vi "oax_gsLoad Shaft Centerline Data.vi"(11 "data type":i32(listbox)) -> (0 "error out":errorcluster, 1 "end position":i32, 2 "current position":i32, 3 "refnum":refnum<file>, 4 "channel info":T1[](array[typedef]) {"pregain" format="%.2f"; "weighting filter" items=["Linear", "A-weighting", "B-weighting", "C-weighting", "ITU-R 468-4", "Dolby", "CCITT", "C-message", "Wb", "Wc", "Wd", "We", "Wf", "Wh", "Wj", "Wk", "Wm", "AES17 20 kHz lowpass", "AES17 40 kHz lowpass", "AES17 20 kHz highpass", "AES17 40 kHz highpass"]; "dB reference" format="%^.1e"; "engineering units" items=["custom..."=0, "V"=1, "A"=21, "C"=30, "pC"=31, "s"=32, "-"=29, "Pa"=2, "N"=20, "g"=3, "m/s^2"=4, "m/s"=5, "m"=6, "mm/s"=12, "mm"=13, "micron/s"=14, "micron"=15, "in/s^2"=7, "in/s"=8, "in"=9, "mil/s"=10, "mil"=11, "rad/s^2"=16, "rad/s"=17, "rad"=18, "deg/s^2"=26, "deg/s"=27, "deg"=28, "RPM"=22, "cycle/s^2"=23, "Hz"=24, "cycle"=25, "strain"=19]; "sensor sensitivity" format="%#_5f"}, 5 "channel name":string[](array[string]), 6 "pulse / rev":i32)   [LabVIEW 2017]
uses:
  <vilib>/addons/_NISVFA/_Shared subVIs/Controls/svc_Channel Info.ctl
  <vilib>/addons/_NISVFA/_Shared subVIs/Controls/svc_Engineering Units Text Ring.ctl
  <vilib>/addons/_NISVFA/_Shared subVIs/Controls/svc_Weighting Filter Text Ring.ctl
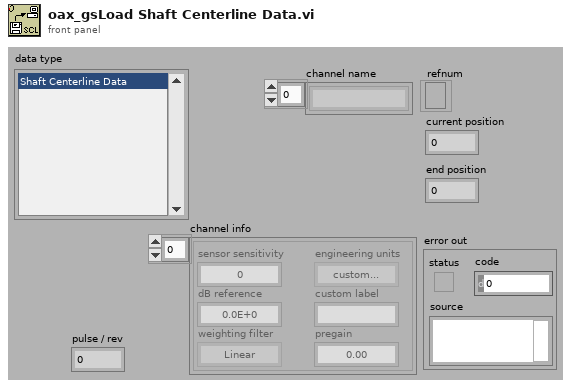
[diagram p1: front panel]
types:
  T1 = typedef "svc_Channel Info.ctl" = cluster{"sensor sensitivity":dbl, "engineering units":T2, "dB reference":dbl, "custom label":string, "weighting filter":T3, "pregain":dbl}
  T2 = typedef "svc_Engineering Units Text Ring.ctl" = u16
  T3 = typedef "svc_Weighting Filter Text Ring.ctl" = u16
  T4 = enum16{"open", "open or create", "create or replace", "create", "open (read only)"}
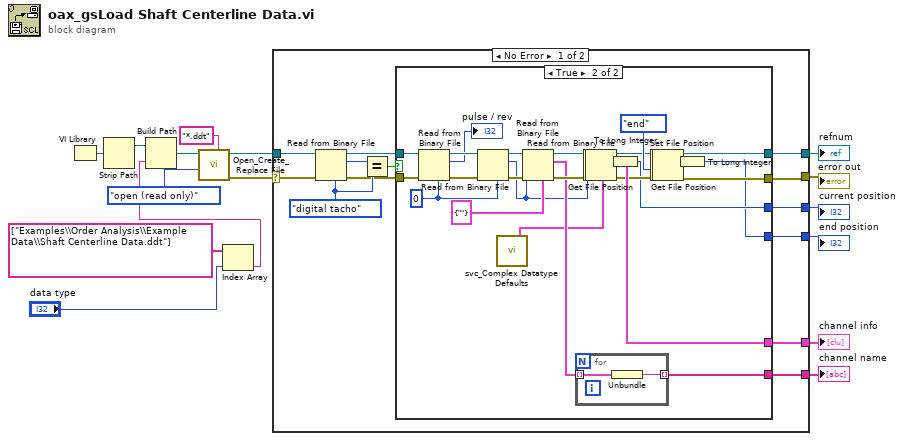
[diagram p0: block diagram]
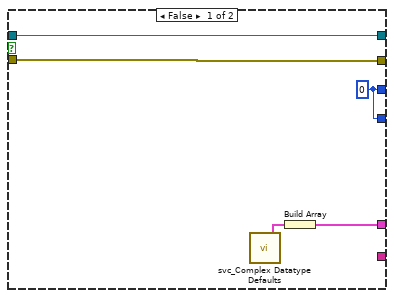
[diagram p2: hidden frame]
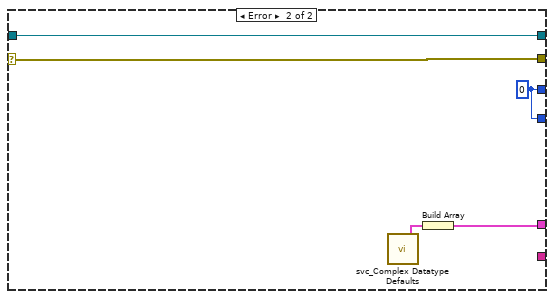
[diagram p3: hidden frame]
diagram:
  n1 = VI Library() -> (path=w14:path)
  n2 = Strip Path(path=w14) -> (stripped path=w13:path)  [unwired: 1 out]
  n3 = Index Array(array=string[] ["Examples\\Order Analysis\\Example Data\\Shaft Centerline Data.ddt"], index="data type") -> (element=w1:string)
  n4 = Build Path(base path=w13, name or relative path=w1) -> (appended path=w12:path)
  n5 = call <vilib>:"Open_Create_Replace File.vi"("pattern"="*.ddt", "function (open:0)"=T4."open (read only)", "file path"=w12) -> ("error out"=w10:errorcluster, "refnum"=w11:refnum<file>)  [unwired: 5 in, 2 out]
  n6 = case shown="No Error" w10 {
    selector: w10 -> [w25 w70]
    tunnel: [w19 w70] -> w8
    tunnel: w11 -> [w29 w69]
    tunnel: [w20 w69] -> w9
    tunnel: [w22 w67] -> w5
    tunnel: [w21 _] -> w4
    tunnel: [w18 w66] -> w7
    tunnel: [w17 w66] -> w6
    frame No Error {
      w27 = enum16{"analog tacho", "digital tacho"}."digital tacho"
      n7 = Read from Binary File(5:w27, 8:w25, 11:w29) -> (0:w23:errorcluster, 2:w28:enum16{"analog tacho", "digital tacho"}, 3:w24:refnum<file>)  [unwired: 3 in, 1 out]
      n8 = Equal?(x=w28, y=w27) -> (x = y?=w26:bool)
      n9 = case shown="True" w26 {
        tunnel: w24 -> [w34 w62]
        tunnel: w23 -> [w33 w63]
        tunnel: [w31 w51] -> w22
        tunnel: [_ w55] -> w21
        tunnel: [w34 w44] -> w20
        tunnel: [w33 w43] -> w19
        tunnel: [w30 w42] -> w18
        tunnel: [w30 w41] -> w17
        frame False {
          w30 = 0 ("offset")
          n10 = call <vilib>:"svc_Complex Datatype Defaults.vi"() -> ("channel info"=w32:T1)  [unwired: 11 in, 8 out]
          n11 = Build Array(w32) -> (w31:T1[])
        }
        frame True {
          w50 = 0
          n12 = Read from Binary File(5:w50, 8:w63, 11:w62) -> (0:w59:errorcluster, 2:→"pulse / rev":i32, 3:w57:refnum<file>)  [unwired: 3 in, 1 out]
          n13 = Read from Binary File(5:w50, 8:w59, 11:w57) -> (0:w58:errorcluster, 2:w48:i32, 3:w56:refnum<file>)  [unwired: 3 in, 1 out]
          n14 = call <vilib>:"svc_Complex Datatype Defaults.vi"() -> ("channel info"=w45:T1)  [unwired: 11 in, 8 out]
          n15 = Read from Binary File(5:cluster{"ch0 string":string} {"ch0 string"=""}, 8:w58, 10:w48, 11:w56) -> (0:w61:errorcluster, 2:w52:cluster{"ch0 string":string}[], 3:w60:refnum<file>)  [unwired: 2 in, 1 out]
          n16 = for {
            tunnel: w52 -> [w65] mode=indexing
            tunnel: [w64] -> w55 mode=indexing
            n17 = Unbundle(w65) -> ("ch0 string"=w64:string)
          }
          n18 = Read from Binary File(5:w45, 8:w61, 10:w48, 11:w60) -> (0:w36:errorcluster, 2:w51:T1[], 3:w37:refnum<file>)  [unwired: 2 in, 1 out]
          n19 = Get File Position(4:w36, 7:w37) -> (0:w47:errorcluster, 2:w35:i64, 3:w46:refnum<file>)
          n20 = To Long Integer(number=w35) -> (32bit integer=w42:i32)
          n21 = Set File Position(refnum=w46, from (0:start)=enum16{"start", "end", "current"}."end" ("pos mode (0:2)"), error in=w47) -> (refnum out=w40:refnum<file>, error out=w39:errorcluster)  [unwired: 1 in]
          n22 = Get File Position(4:w39, 7:w40) -> (0:w43:errorcluster, 2:w38:i64, 3:w44:refnum<file>)
          n23 = To Long Integer(number=w38) -> (32bit integer=w41:i32)
        }
      }
    }
    frame Error {
      w66 = 0 ("offset")
      n24 = call <vilib>:"svc_Complex Datatype Defaults.vi"() -> ("channel info"=w68:T1)  [unwired: 11 in, 8 out]
      n25 = Build Array(w68) -> (w67:T1[])
    }
  }
  "refnum" <- w9
  "error out" <- w8
  "current position" <- w7
  "end position" <- w6
  "channel info" <- w5
  "channel name" <- w4
